vi "Get Wire Data Type.vi"(8 "error in (no error)":errorcluster, 11 "Wire ref in":refnum<vi>) -> (0 "error out":errorcluster, 2 "Type":T1, 3 "Wire ref out":refnum<vi>)   [LabVIEW 2016]
uses:
  <vilib>/Utility/Data Type/Type Definitions/Data Type.ctl
  <vilib>/Utility/Data Type/NI_Data Type.lvlib
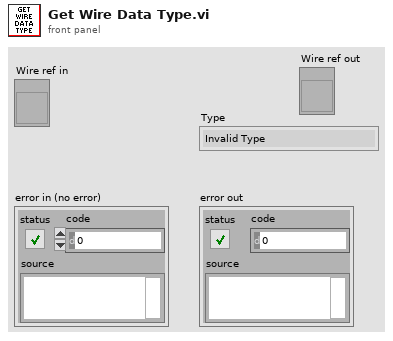
[diagram p1: front panel]
types:
  T1 = typedef "NI_Data Type.lvlib/Data Type.ctl" = enum8{"Invalid Type", "Void", "I8", "I16", "I32", "I64", "U8", "U16", "U32", "U64", "Single Float", "Double Float", "Extended Float", "Single Complex", "Double Complex", "Extended Complex", "Enum U8", "Enum U16", "Enum U32", "Enum U64", "Single Float With Unit", "Double Float With Unit", "Extended Float With Unit", "Single Complex with Unit", "Double Complex with Unit", "Extended Complex with Unit", "Boolean", "String", "Path", "Picture", "Tag", "Array", "Cluster", "Variant", "LV Variant", "Waveform", "Timestamp", "Digital Waveform", "Digital Data", "ExpressData", "Refnum", "External Data", "VI", "Poly VI", "LabVIEW Class Instance", "Fixed Point"}
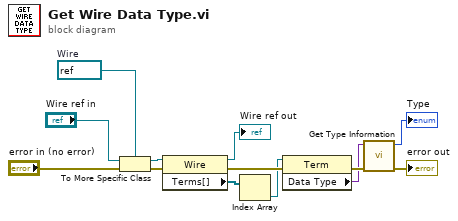
[diagram p0: block diagram]
diagram:
  w4 = refnum<vi> refnum  # Wire
  n1 = To More Specific Class(target class=w4, reference="Wire ref in", error in="error in (no error)") -> (specific class reference=w5:refnum<vi>, error out=w6:errorcluster)
  n2 = property class="Wire"(reference=w5, error in=w6) -> (reference out=→"Wire ref out":refnum<vi>, error out=w10:errorcluster, "Terms[]"=w7:refnum<vi>[])
  n3 = Index Array(array=w7) -> (element=w9:refnum<vi>)  [unwired: 1 in]
  n4 = property class="Term"(reference=w9, error in=w10) -> (error out=w11:errorcluster, "Data Type"=w8:variant)  [unwired: 1 out]
  n5 = call <vilib>:"Get Type Information.vi"("error in (no error)"=w11, "Variant"=w8) -> ("error out"=→"error out":errorcluster, "Type"=→"Type":T1)  [unwired: 5 in, 3 out]
